vi "Periodic Tasks.vi"(8 "error in":errorcluster) -> ()   [LabVIEW 2016]
doc: "This VI runs in parallel to other tasks. It can contain as many user-defined periodic loops as you need. These can carry out PID or other sorts of timed response."
uses:
  <vilib>/Rock Robotics/WPI/Relay/WPI_RelayValue.ctl
  <vilib>/Rock Robotics/WPI/Utilities/WPI_GetSetVariantRefNum.vi
  Robot Global Data.vi
panel:
  out "RelayValue":T1
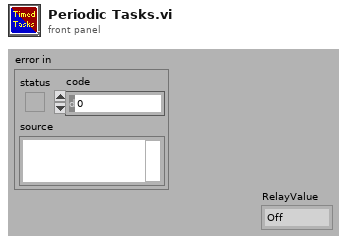
[diagram p1: front panel]
types:
  T1 = typedef "WPI_RelayValue.ctl" = enum16{"Off", "On", "Forward", "Reverse"}
  T2 = typedef "WPI_JoystickDevRef.ctl" = cluster{"Device":T3}
  T3 = typedef "WPI_JoystickDeviceEnum.ctl" = enum16{"USB 0", "USB 1", "USB 2", "USB 3", "USB 4", "USB 5"}
  T4 = typedef "WPI_RobotDriveDevRef.ctl" = cluster{"DevStatus":errorcluster, "Motors[]":T5[], "Square Inputs":bool, "Max Output":dbl}
  T5 = typedef "WPI_MotorControlDeviceRef.ctl" = cluster{"DeviceStatus":errorcluster, "Type":T6, "PWM":cluster{"PWM Channel":T7, "DeadBand":T8}, "CAN":cluster{"Device Number":u8, "SetOutput VI Ref":variant, "GetOutput VI Ref":variant, "Enable VI Ref":variant, "Disable VI Ref":variant, "Data":variant}, "Invert":bool}
  T6 = typedef "WPI_MotorControlType.ctl" = enum16{"PWM", "CAN"}
  T7 = typedef "FPGA_DIOPWMChannel.ctl" = enum8{"PWM 0", "PWM 1", "PWM 2", "PWM 3", "PWM 4", "PWM 5", "PWM 6", "PWM 7", "PWM 8", "PWM 9", "PWM MXP 0", "PWM MXP 1", "PWM MXP 2", "PWM MXP 3", "PWM MXP 4", "PWM MXP 5", "PWM MXP 6", "PWM MXP 7", "PWM MXP 8", "PWM MXP 9", "Invalid"}
  T8 = typedef "WPI_PWMDeadband.ctl" = cluster{"Name":string, "maxPositivePwm":i32, "minPositivePwm":i32, "centerPwm":i32, "maxNegativePwm":i32, "minNegativePwm":i32, "angularRange":u16}
  T9 = typedef "WPI_RelayDevRef.ctl" = cluster{"DevStatus":errorcluster, "Relay Channel":T10, "Relay Direction":T11}
  T10 = typedef "FPGA_DIORelayChannel.ctl" = enum8{"Relay 0", "Relay 1", "Relay 2", "Relay 3", "Invalid"}
  T11 = typedef "WPI_RelayDirection.ctl" = enum16{"Both directions", "Forward only", "Reverse only"}
  T12 = cluster{"JoystickDevRef":T2, "RobotDriveDevRef":T4}
  T13 = cluster{"Current Gear":enum16{"Low", "High"}, "Gear Shift State":enum16{"Low", "Shifting", "High"}}
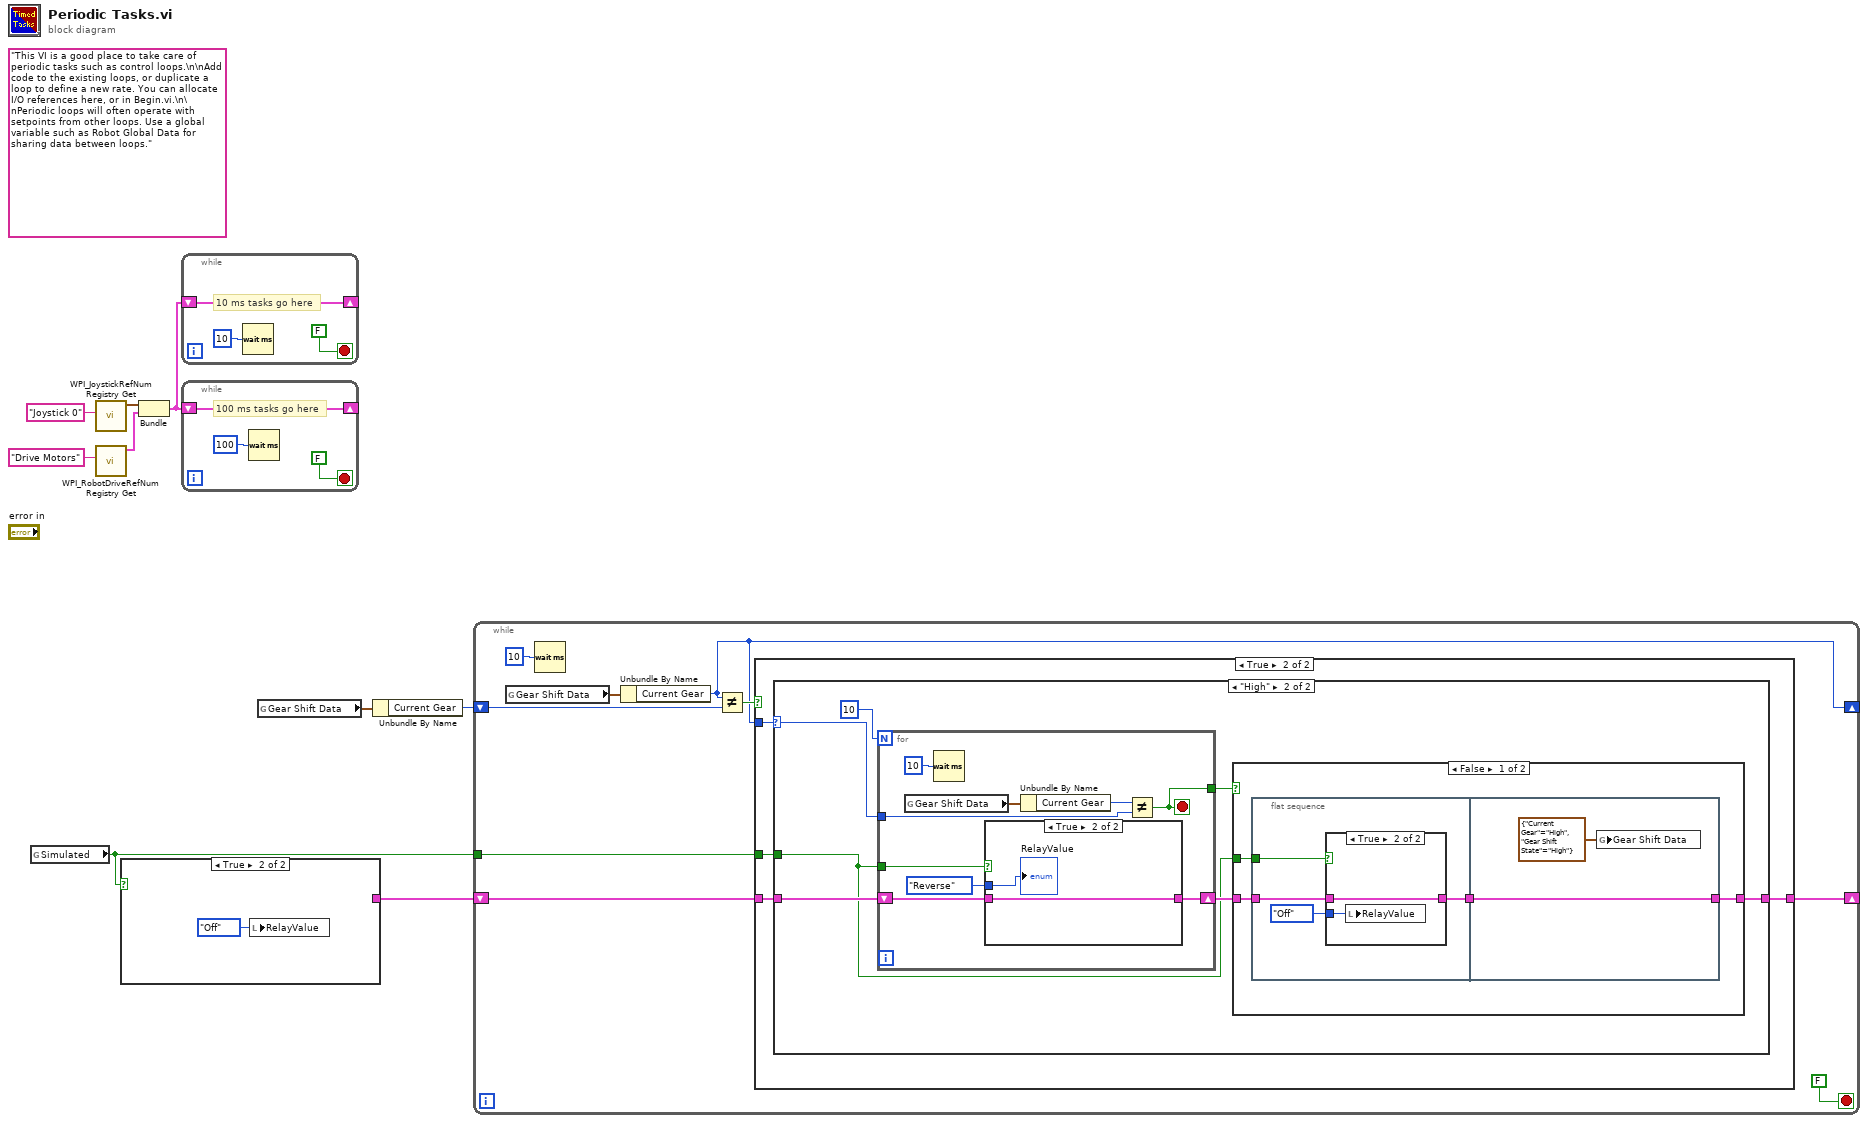
[diagram p0: block diagram]
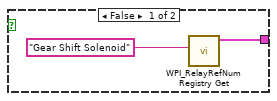
[diagram p2: hidden frame]
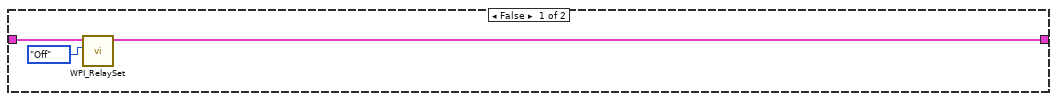
[diagram p3: hidden frame]
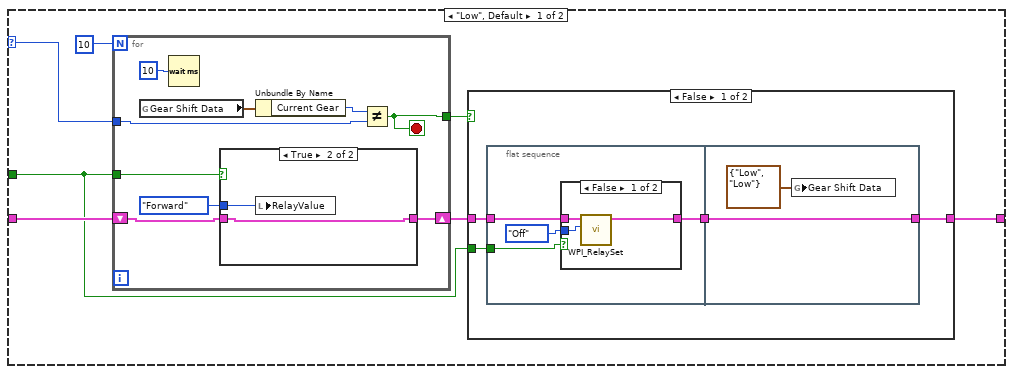
[diagram p4: hidden frame]
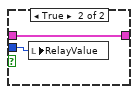
[diagram p5: hidden frame]
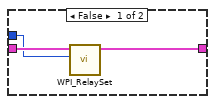
[diagram p7: hidden frame]
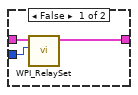
[diagram p8: hidden frame]
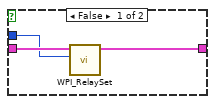
[diagram p10: hidden frame]
diagram:
  (unwired) "This VI is a good place to take care of periodic tasks such as control loops.\n\nAdd code to the existing loops, or duplicate a loop to define a new rate. You can allocate I/O references here, or in Begin.vi.\n\nPeriodic loops will often operate with setpoints from other loops. Use a global variable such as Robot Global Data for sharing data between loops."
  n1 = global read "Robot Global Data.vi" "Simulated"() -> (w1:bool)
  n2 = call <vilib>:"WPI_JoystickRefNum Registry Get.vi"("refnum name"="Joystick 0") -> ("JoystickDevRef"=w7:T2)  [unwired: 1 in, 9 out]
  n3 = call <vilib>:"WPI_RobotDriveRefNum Registry Get.vi"("refnum name"="Drive Motors") -> ("RobotDriveDevRef"=w6:T4)  [unwired: 1 in, 9 out]
  n4 = case shown="True" w1 {
    tunnel: [w10 _] -> w2
    frame False {
      n5 = call <vilib>:"WPI_RelayRefNum Registry Get.vi"("refnum name"="Gear Shift Solenoid") -> ("RelayDevRef"=w10:T9)  [unwired: 9 in, 1 out]
    }
    frame True {
      n6 = local write "RelayValue"(WPI_RelayValue."Off" ("RelayValue")) -> ()
    }
  }
  n7 = Bundle("JoystickDevRef"=w7, "RobotDriveDevRef"=w6) -> (w5:T12)  [unwired: 1 out]
  n8 = while {
    shift-right: [w13] -> _
    shift-left: w5 -> [w13]
    stop <- FALSE stop-if-true
    # "10 ms tasks go here"
    n9 = Wait (ms)(milliseconds to wait=u32 10) -> ()  [unwired: 1 out]
  }
  n10 = while {
    shift-right: [w16] -> _
    shift-left: w5 -> [w16]
    stop <- FALSE stop-if-true
    # "100 ms tasks go here"
    n11 = Wait (ms)(milliseconds to wait=u32 100) -> ()  [unwired: 1 out]
  }
  n12 = global read "Robot Global Data.vi" "Gear Shift Data"() -> (w4:T13)
  n13 = Unbundle By Name(w4) -> ("Current Gear"=w3:enum16{"Low", "High"})
  n14 = while {
    shift-right: [w22] -> _
    shift-left: w3 -> [w24]
    shift-right: [w20] -> _
    shift-left: w2 -> [w21]
    tunnel: w1 -> [w19]
    stop <- FALSE stop-if-true
    n15 = global read "Robot Global Data.vi" "Gear Shift Data"() -> (w25:T13)
    n16 = Wait (ms)(milliseconds to wait=u32 10) -> ()  [unwired: 1 out]
    n17 = Unbundle By Name(w25) -> ("Current Gear"=w22:enum16{"Low", "High"})
    n18 = Not Equal?(x=w22, y=w24) -> (x != y?=w23:bool)
    n19 = case shown="True" w23 {
      tunnel: w22 -> [_ w34]
      tunnel: w21 -> [w30 w33]
      tunnel: [w28 w32] -> w20
      tunnel: w19 -> [_ w31]
      frame False {
        n20 = call <vilib>:"WPI_RelaySet.vi"("RelayValue"=WPI_RelayValue."Off", "RelayDevRef"=w30) -> ("RelayDevRef"=w28:T9)  [unwired: 8 in, 1 out]
      }
      frame True {
        n21 = case shown="\"High\"" w34 {
          selector: w34 -> [w40 w76]
          tunnel: w33 -> [w41 w75]
          tunnel: [w39 w74] -> w32
          tunnel: w31 -> [w35 w72]
          frame "Low", Default {
            n22 = for {
              N: 10 -> [_]
              shift-right: [w64] -> w38
              shift-left: w41 -> [w66]
              tunnel: w40 -> [w61]
              tunnel: [w59] -> w36
              tunnel: w35 -> [w58]
              stop <- w59 stop-if-true
              n23 = global read "Robot Global Data.vi" "Gear Shift Data"() -> (w63:T13)
              n24 = Wait (ms)(milliseconds to wait=u32 10) -> ()  [unwired: 1 out]
              n25 = case shown="True" w58 {
                tunnel: w66 -> [w69 w71]
                tunnel: WPI_RelayValue."Forward" ("RelayValue") -> [w68 w70]
                tunnel: [w67 w71] -> w64
                frame False {
                  n26 = call <vilib>:"WPI_RelaySet.vi"("RelayValue"=w68, "RelayDevRef"=w69) -> ("RelayDevRef"=w67:T9)  [unwired: 8 in, 1 out]
                }
                frame True {
                  n27 = local write "RelayValue"(w70) -> ()
                }
              }
              n28 = Unbundle By Name(w63) -> ("Current Gear"=w62:enum16{"Low", "High"})
              n29 = Not Equal?(x=w62, y=w61) -> (x != y?=w59:bool)
            }
            n30 = case shown="False" w36 {
              tunnel: [w44 w57] -> w39
              tunnel: w38 -> [w43 w57]
              tunnel: w35 -> [w42 _]
              frame False {
                n31 = flat-sequence {
                  tunnel: w43 -> [w49]
                  tunnel: [w48] -> w45
                  tunnel: w42 -> [w46]
                  tunnel: [w56] -> w44
                  tunnel: w45 -> [w56]
                  frame #0 {
                    n32 = case shown="False" w46 {
                      tunnel: w49 -> [w52 w54]
                      tunnel: [w51 w54] -> w48
                      tunnel: WPI_RelayValue."Off" ("RelayValue") -> [w50 w53]
                      frame False {
                        n33 = call <vilib>:"WPI_RelaySet.vi"("RelayValue"=w50, "RelayDevRef"=w52) -> ("RelayDevRef"=w51:T9)  [unwired: 8 in, 1 out]
                      }
                      frame True {
                        n34 = local write "RelayValue"(w53) -> ()
                      }
                    }
                  }
                  frame #1 {
                    n35 = global write "Robot Global Data.vi" "Gear Shift Data"(T13 {"Current Gear"=enum."Low", "Gear Shift State"=enum."Low"} ("Gear Shift Data")) -> ()
                  }
                }
              }
              frame True {
              }
            }
          }
          frame "High" {
            n36 = for {
              N: 10 -> [_]
              shift-right: [w102] -> w78
              shift-left: w75 -> [w103]
              tunnel: w76 -> [w99]
              tunnel: [w97] -> w73
              tunnel: w72 -> [w96]
              stop <- w97 stop-if-true
              n37 = global read "Robot Global Data.vi" "Gear Shift Data"() -> (w101:T13)
              n38 = Wait (ms)(milliseconds to wait=u32 10) -> ()  [unwired: 1 out]
              n39 = case shown="True" w96 {
                tunnel: w103 -> [w106 w107]
                tunnel: [w105 w107] -> w102
                tunnel: WPI_RelayValue."Reverse" ("RelayValue") -> [w104 w108]
                frame False {
                  n40 = call <vilib>:"WPI_RelaySet.vi"("RelayValue"=w104, "RelayDevRef"=w106) -> ("RelayDevRef"=w105:T9)  [unwired: 8 in, 1 out]
                }
                frame True {
                  "RelayValue" <- w108
                }
              }
              n41 = Unbundle By Name(w101) -> ("Current Gear"=w100:enum16{"Low", "High"})
              n42 = Not Equal?(x=w100, y=w99) -> (x != y?=w97:bool)
            }
            n43 = case shown="False" w73 {
              tunnel: w78 -> [w81 w94]
              tunnel: [w80 w94] -> w74
              tunnel: w72 -> [w79 _]
              frame False {
                n44 = flat-sequence {
                  tunnel: w81 -> [w86]
                  tunnel: [w85] -> w82
                  tunnel: w79 -> [w83]
                  tunnel: [w93] -> w80
                  tunnel: w82 -> [w93]
                  frame #0 {
                    n45 = case shown="True" w83 {
                      tunnel: w86 -> [w89 w91]
                      tunnel: [w88 w91] -> w85
                      tunnel: WPI_RelayValue."Off" ("RelayValue") -> [w87 w90]
                      frame False {
                        n46 = call <vilib>:"WPI_RelaySet.vi"("RelayValue"=w87, "RelayDevRef"=w89) -> ("RelayDevRef"=w88:T9)  [unwired: 8 in, 1 out]
                      }
                      frame True {
                        n47 = local write "RelayValue"(w90) -> ()
                      }
                    }
                  }
                  frame #1 {
                    n48 = global write "Robot Global Data.vi" "Gear Shift Data"(T13 {"Current Gear"=enum."High", "Gear Shift State"=enum."High"} ("Gear Shift Data")) -> ()
                  }
                }
              }
              frame True {
              }
            }
          }
        }
      }
    }
  }
